vi "Map Collection - Comparing Test Results_Generate.vi"() -> (2 "measurement event refnum":refnum<user-event>, 3 "registration refnum":refnum<event-registration>)   [LabVIEW 2023]
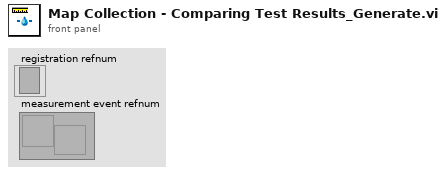
[diagram p1: front panel]
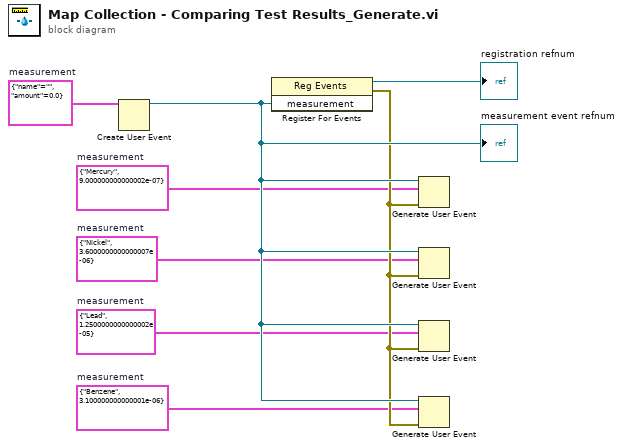
[diagram p0: block diagram]
diagram:
  w6 = cluster{"name":string, "amount":dbl[unit]} {"name"="Benzene", "amount"=3.100000000000001e-06}  # measurement
  w5 = cluster{"name":string, "amount":dbl[unit]} {"name"="Lead", "amount"=1.2500000000000002e-05}  # measurement
  w4 = cluster{"name":string, "amount":dbl[unit]} {"name"="Nickel", "amount"=3.6000000000000007e-06}  # measurement
  w3 = cluster{"name":string, "amount":dbl[unit]} {"name"="Mercury", "amount"=9.000000000000002e-07}  # measurement
  w2 = cluster{"name":string, "amount":dbl[unit]} {"name"="", "amount"=0.0}  # measurement
  n1 = Create User Event(user event datatype=w2) -> (user event=w8:refnum<user-event>)  [unwired: 1 in, 1 out]
  "measurement event refnum" <- w8
  n2 = register-events(w8) -> (reference out=→"registration refnum":refnum<event-registration>, error out=w7:errorcluster)  [unwired: 2 in]
  n3 = Generate User Event(user event=w8, event data cluster=w3, error in=w7) -> ()  [unwired: 1 in, 2 out]
  n4 = Generate User Event(user event=w8, event data cluster=w4, error in=w7) -> ()  [unwired: 1 in, 2 out]
  n5 = Generate User Event(user event=w8, event data cluster=w5, error in=w7) -> ()  [unwired: 1 in, 2 out]
  n6 = Generate User Event(user event=w8, event data cluster=w6, error in=w7) -> ()  [unwired: 1 in, 2 out]
